vi "CheeseReciveGeneric.vi"() -> (2 "Right Hot":bool, 3 "Left Hot":bool)   [LabVIEW 2013]
uses:
  TCPServerStates.ctl
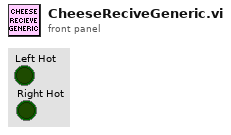
[diagram p1: front panel]
types:
  T1 = typedef "TCPServerStates.ctl" = enum16{"Listening", "Connected"}
  T2 = enum16{"Standard", "Buffered", "CRLF", "Immediate"}
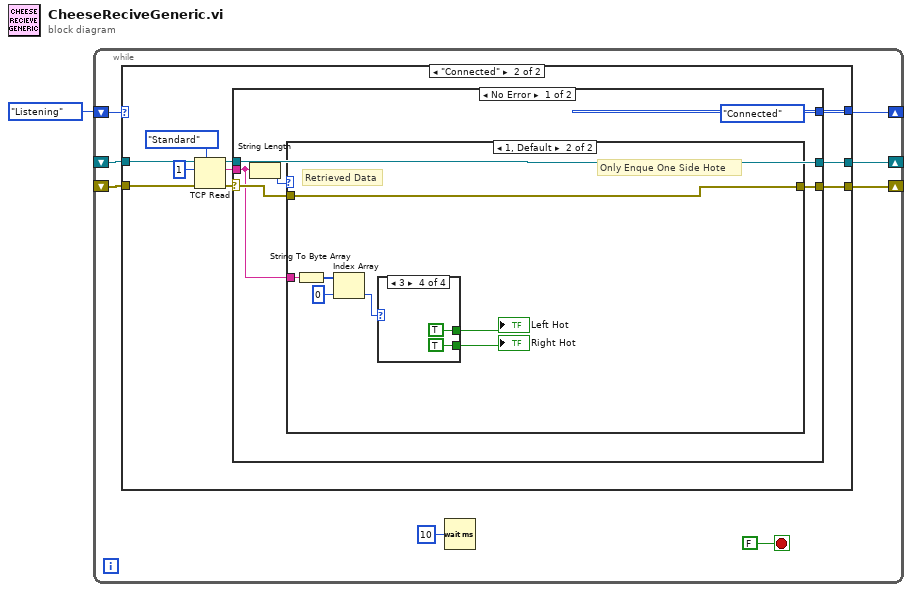
[diagram p0: block diagram]
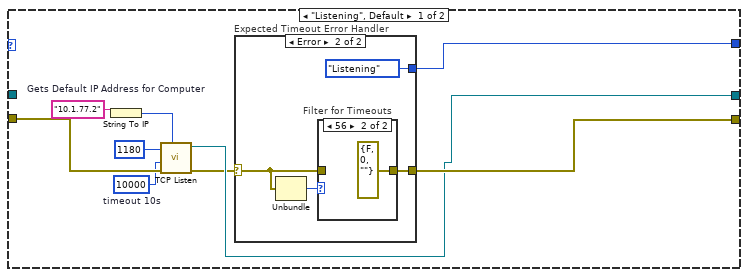
[diagram p2: hidden frame]
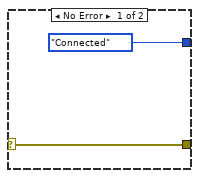
[diagram p3: hidden frame]
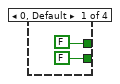
[diagram p6: hidden frame]
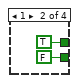
[diagram p7: hidden frame]
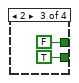
[diagram p8: hidden frame]
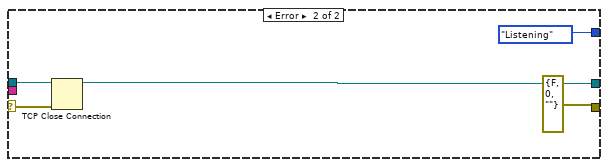
[diagram p9: hidden frame]
diagram:
  n1 = while {
    shift-right: [w7] -> _
    shift-left: _ -> [w5]
    shift-right: [w6] -> _
    shift-left: TCPServerStates."Listening" -> [w8]
    shift-right: [w4] -> _
    shift-left: _ -> [w3]
    stop <- FALSE stop-if-true
    n2 = case shown="\"Connected\"" w8 {
      tunnel: [w18 w33] -> w7
      tunnel: [w17 w32] -> w6
      tunnel: w5 -> [w16 w36]
      tunnel: [w15 w34] -> w4
      tunnel: w3 -> [_ w35]
      frame "Listening", Default {
        w14 = 10000  # timeout 10s
        n3 = String To IP "Gets Default IP Address for Computer"(1:"10.1.77.2" ("name")) -> (0:w11:u32)
        n4 = call <vilib>:"TCP Listen.vi"("net address"=w11, "error in (no error)"=w16, "timeout ms (wait forever: -1)"=w14, "port"=u16 1180) -> ("error out"=w12:errorcluster, "connection ID"=w15:refnum<k5>)  [unwired: 3 in, 3 out]
        n5 = case "Expected Timeout Error Handler" shown="Error" w12 {
          selector: w12 -> [w20 w22]
          tunnel: [w20 w23] -> w18
          tunnel: [TCPServerStates."Connected" TCPServerStates."Listening"] -> w17
          frame No Error {
          }
          frame Error {
            n6 = Unbundle(w22) -> ("code"=w24:i32)  [unwired: 2 out]
            n7 = case "Filter for Timeouts" shown="56" w24 {
              tunnel: [w25 errorcluster {"status"=FALSE, "code"=0, "source"=""} ("error constant")] -> w23
              tunnel: w22 -> [w25 _]
              frame 0, Default {
              }
              frame 56 {
              }
            }
          }
        }
      }
      frame "Connected" {
        n8 = TCP Read(connection ID=w35, bytes to read=1, error in (no error)=w36, 7:T2."Standard" ("mode (standard)")) -> (connection ID out=w28:refnum<k5>, data out=w30:string, error out=w29:errorcluster)  [unwired: 1 in]
        n9 = case shown="No Error" w29 {
          selector: w29 -> [w40 w59]
          tunnel: w30 -> [w37 _]
          tunnel: w28 -> [w41 w61]
          tunnel: [w41 w60] -> w34
          tunnel: [w39 errorcluster {"status"=FALSE, "code"=0, "source"=""} ("error IO")] -> w33
          tunnel: [TCPServerStates."Connected" TCPServerStates."Listening"] -> w32
          frame No Error {
            n10 = String Length(string=w37) -> (length=w42:i32)
            n11 = case shown="1, Default" w42 {
              tunnel: w40 -> [w43 w44]
              tunnel: [w43 w44] -> w39
              tunnel: w37 -> [_ w50]
              frame 0 {
                # "No Data"
              }
              frame 1, Default {
                # "Only Enque One Side Hote"
                # "Retrieved Data"
                n12 = String To Byte Array(string=w50) -> (unsigned byte array=w49:u8[])
                n13 = Index Array(array=w49, index=0) -> (element=w45:u8)
                n14 = case shown="3" w45 {
                  tunnel: [FALSE ("Left Hot") TRUE ("Left Hot") FALSE ("Left Hot") TRUE ("Left Hot")] -> w46
                  tunnel: [FALSE ("Left Hot") FALSE ("Left Hot") TRUE ("Left Hot") TRUE ("Left Hot")] -> w47
                  frame 0, Default {
                  }
                  frame 1 {
                  }
                  frame 2 {
                  }
                  frame 3 {
                  }
                }
                "Left Hot" <- w46
                "Right Hot" <- w47
              }
            }
          }
          frame Error {
            n15 = TCP Close Connection(connection ID=w61, error in (no error)=w59) -> (connection ID out=w60:refnum<k5>)  [unwired: 1 in, 1 out]
          }
        }
      }
    }
    n16 = Wait (ms)(milliseconds to wait=u32 10) -> ()  [unwired: 1 out]
  }
